vi "RS232.vi"(1 "Command":string="VDC;\nAUTO;*TRG;RWLS;RATE F\n", 2 "VISA资源名称":refnum<visa-resource-name>="COM20") -> (0 "响应":string)   [LabVIEW 2015]
doc: "本范例执行串口读写操作。串口设置的参数必须匹配连接仪器或设备的参数。“VISA配置串口”VI可设置配置参数。前面板显示的控件可用于配置基本参数，如波特率、数据位和校验。VI会将VISA资源名称传递至其他VI以便执行相关操作。“VISA写入”函数将发送一个命令至串行设备，“VISA读取”函数将返回基于该命令的数据。“VISA关闭”函数可关闭该串行设备的引用。关闭引用十分重要，否则可能导致无法通过该端口进行进一步通信。"
uses:
  Serial - Settings.ctl
  <vilib>/Instr/_visa.llb/VISA Configure Serial Port (Instr).vi
panel:
  in  "串口设置":T1={"波特率"=9600, "数据比特"=8, "奇偶"=enum."None", "停止位"=10, "流控制"=0} {"流控制" items=["无"=0, "XON/XOFF"=1, "RTS/CTS"=2, "DTR/DSR"=4]; "停止位" items=["1.0"=10, "1.5"=15, "2.0"=20]; "数据比特" min=5 max=8 step=1; "波特率" items=["75"=75, "110"=110, "134"=134, "150"=150, "300"=300, "600"=600, "1200"=1200, "1800"=1800, "2400"=2400, "4800"=4800, "7200"=7200, "9600"=9600, "14400"=14400, "19200"=19200, "28800"=28800, "38400"=38400, "56000"=56000, "57600"=57600, "115200"=115200, "128000"=128000, "230400"=230400]}
  out "读取的字节":u32
  in  "读取前延时(ms)":u32=500
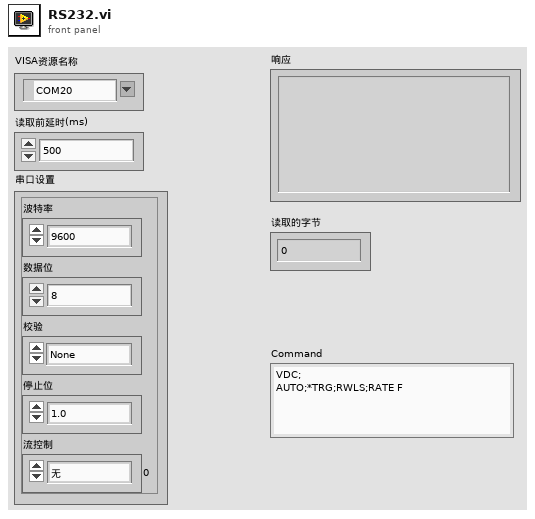
[diagram p1: front panel]
types:
  T1 = typedef "Serial - Settings.ctl" = cluster{"波特率":u32, "数据比特":u16, "奇偶":enum16{"None", "Odd", "Even", "Mark", "Space"}, "停止位":u16, "流控制":u16}
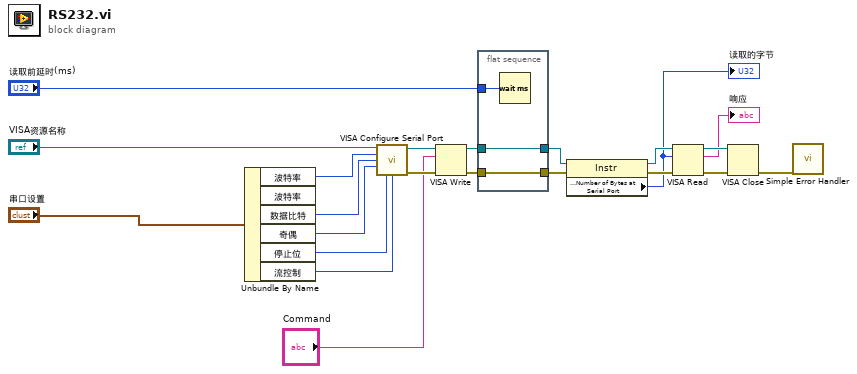
[diagram p0: block diagram]
diagram:
  n1 = Unbundle By Name("串口设置") -> ("波特率"=w7:u32, "数据比特"=w6:u16, "奇偶"=w5:enum16{"None", "Odd", "Even", "Mark", "Space"}, "停止位"=w4:u16, "流控制"=w3:u16)  [unwired: 1 out]
  n2 = call-poly "VISA Configure Serial Port"("VISA resource name"="VISA资源名称", "baud rate (9600)"=w7, "data bits (8)"=w6, "parity (0:none)"=w5, "stop bits (10: 1 bit)"=w4, "flow control (0:none)"=w3) -> ("VISA resource name out"=w20:refnum<visa-resource-name>, "error out"=w21:errorcluster)  [unwired: 3 in, 5 out]
  n3 = VISA Write(VISA resource name=w20, write buffer="Command", error in (no error)=w21) -> (VISA resource name out=w15:refnum<visa-resource-name>, error out=w17:errorcluster)  [unwired: 1 out]
  n4 = flat-sequence {
    tunnel: w17 -> [w24]
    tunnel: [w24] -> w16
    tunnel: w15 -> [w23]
    tunnel: [w23] -> w14
    tunnel: "读取前延时(ms)" -> [w25]
    frame #0 {
      n5 = Wait (ms)(milliseconds to wait=w25) -> ()  [unwired: 1 out]
    }
  }
  n6 = property class="Instr"(reference=w14, error in=w16) -> (reference out=w11:refnum<visa-resource-name>, error out=w10:errorcluster, "Serial Settings:Number of Bytes at Serial Port"=w1:u32)
  "读取的字节" <- w1
  n7 = VISA Read(VISA resource name=w11, byte count=w1, error in (no error)=w10) -> (VISA resource name out=w18:refnum<visa-resource-name>, read buffer=→"响应":string, error out=w19:errorcluster)  [unwired: 1 out]
  n8 = VISA Close(VISA resource name=w18, error in (no error)=w19) -> (error out=w2:errorcluster)
  n9 = call <vilib>:"Simple Error Handler.vi"("error in (no error)"=w2) -> ()  [unwired: 1 in, 8 out]
